vi "Install or Uninstall Components.vi"(4 "Version Selection (Highest)":u32[](array[ring]) items=["Highest", "Exactly"], 6 "Auto-select Dependencies (T)":bool=TRUE, 7 "Restart Automatically (T)":bool=TRUE, 8 "error in (no error)":errorcluster, 9 "Software IDs to Uninstall":string[](array[string]), 10 "Software Components to Install":T2[](array[typedef]) {"component type" items=["standard", "hidden", "system", "unknown", "startup", "image"]}, 11 "Session in":refnum<k21>) -> (0 "error out":errorcluster, 1 "Broken Dependencies":T1[](array[typedef]) {"dependee"."component type" items=["standard", "hidden", "system", "unknown", "startup", "image"]; "depender"."component type" items=["standard", "hidden", "system", "unknown", "startup", "image"]}, 3 "Session out":refnum<k21>)   [LabVIEW 2012, in "nisyscfg.lvlib"]
doc: "Use the Install or Uninstall Components VI to install components, uninstall components, or do both installation and uninstallation at once (as long as two components do not overlap each other).\n\nThis VI installs components you specify in the <B>Software Components to Install</B> parameter, as well as any required hidden components. If <B>Auto-select Dependencies</B> is TRUE, this VI also installs other visible components if they are dependencies of any component you specified to install in the <B>Software Components to Install</B> parameter and they are not already installed on the system. This VI only uninstalls visible components that are specified in the <B>Software IDs to Uninstall</B> parameter."
uses:
  <vilib>/nisyscfg/nisyscfg.lvlib
  <vilib>/nisyscfg/Software 1.2.ctl
  <vilib>/nisyscfg/Component Type.ctl
  <vilib>/nisyscfg/Broken Dependency 1.2.ctl
  <vilib>/Utility/error.llb/Error Cluster From Error Code.vi
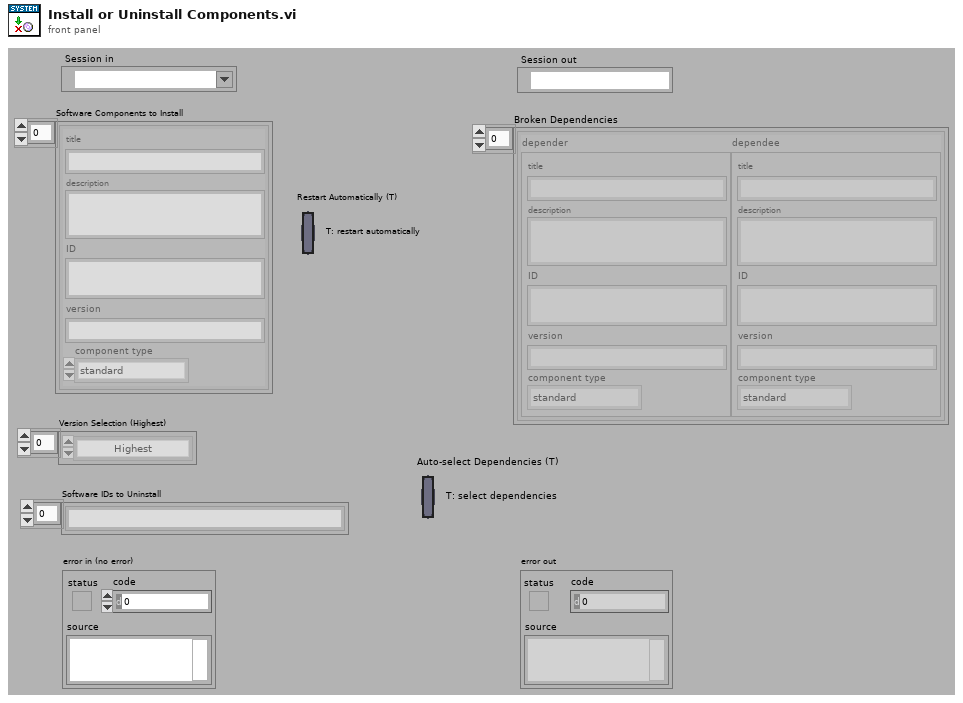
[diagram p1: front panel]
types:
  T1 = typedef "nisyscfg.lvlib/Broken Dependency 1.2.ctl" = cluster{"depender":T2, "dependee":T2}
  T2 = typedef "nisyscfg.lvlib/Software 1.2.ctl" = cluster{"title":string, "description":string, "ID":string, "version":string, "component type":T3}
  T3 = typedef "nisyscfg.lvlib/Component Type.ctl" = u32
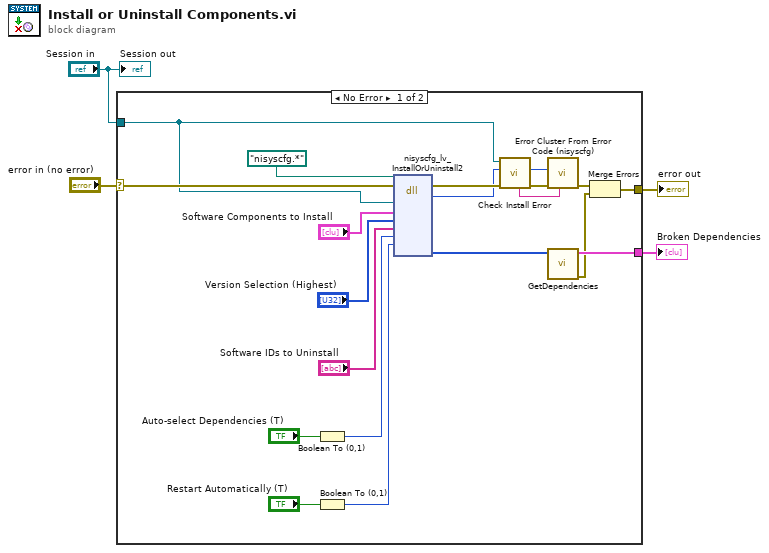
[diagram p0: block diagram]
diagram:
  n1 = case shown="No Error" "error in (no error)" {
    selector: "error in (no error)" -> [w12 w25]
    tunnel: "Session in" -> [w11 _]
    tunnel: [w13 w25] -> w4
    tunnel: [w19 _] -> w3
    frame No Error {
      n2 = Boolean To (0,1)(Boolean="Auto-select Dependencies (T)") -> (0, 1=w21:i16)
      n3 = Boolean To (0,1)(Boolean="Restart Automatically (T)") -> (0, 1=w14:i16)
      n4 = dll-call lib="nisyscfg.*" fn="nisyscfg_lv_InstallOrUninstall2" label="InstallOrUninstall"(path in=path "nisyscfg.*", error in=w12, "session"=w11, "softwareToInstall"="Software Components to Install", "versionSelectionMode"="Version Selection (Highest)", "softwareIDsToUninstall"="Software IDs to Uninstall", "autoSelectDependencies"=w21, "restartAutomatically"=w14) -> (error out=w10:errorcluster, "result"=w9:i32, "brokenDependencies"=w20:u64[])  [unwired: 8 in, 1 out]
      n5 = call <vilib>:"Check Install Error.vi"("error in (no error)"=w10, "Status in"=w9, "Session in"=w11) -> ("error out"=w7:errorcluster, "Status out"=w8:i32, "Details"=w5:string)  [unwired: 5 in, 1 out]
      n6 = call <vilib>:"Error Cluster From Error Code (nisyscfg).vi"("Details String"=w5, "error in (no error)"=w7, "Error Code (0)"=w8) -> ("error out"=w6:errorcluster)  [unwired: 8 in]
      n7 = call <vilib>:"GetDependencies.vi"("Enumerator in"=w20) -> ("error out"=w16:errorcluster, "Dependencies"=w19:T1[])  [unwired: 9 in]
      n8 = Merge Errors(w6, w16) -> (w13:errorcluster)
    }
    frame Error {
    }
  }
  "error out" <- w4
  "Broken Dependencies" <- w3
  "Session out" <- "Session in"
